vi "Test MQTT-3.8.4-5.vi"(8 "error in (no error)":errorcluster, 11 "Connection Config":refnum<class "Connection.lvclass">) -> (0 "error out":errorcluster, 3 "Connection Config dup":refnum<class "Connection.lvclass">)   [LabVIEW 2013]
uses:
  <vilib>/LabVIEW Open Source Project/MQTT Connection/MQTT_Connection/Connection/Connection.lvclass
  <vilib>/LabVIEW Open Source Project/MQTT Control Packets/Control Packets/SUBSCRIBE/Topic Subscription -- cluster.ctl
  <vilib>/LabVIEW Open Source Project/MQTT Control Packets/Control Packets/ControlPacket/QualityOfService -- enum.ctl
  <vilib>/addons/_JKI Toolkits/Caraya/classes/Test/Test.lvclass
  <vilib>/LabVIEW Open Source Project/MQTT Client/Client class/Client.lvclass
  <vilib>/LabVIEW Open Source Project/MQTT Control Packets/Control Packets/SUBSCRIBE/SUBSCRIBE.lvclass
  <vilib>/addons/_JKI Toolkits/Caraya/classes/Assert/Assert.lvclass
  <vilib>/LabVIEW Open Source Project/MQTT Connection/MQTT_Base/Base Class/MQTT_Base.lvclass
  <vilib>/LabVIEW Open Source Project/MQTT Control Packets/Control Packets/ControlPacket/ControlPacket.lvclass
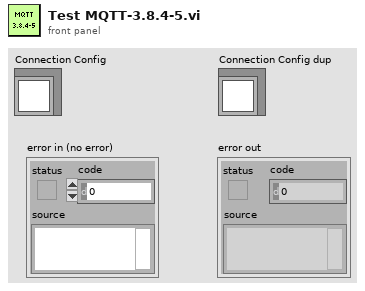
[diagram p1: front panel]
types:
  T1 = typedef "MQTT_Control_Packets.lvlib/SUBSCRIBE.lvclass/Topic Subscription -- cluster.ctl" = cluster{"Topic Filter":string, "QoS":T2}
  T2 = typedef "MQTT_Control_Packets.lvlib/ControlPacket.lvclass/QualityOfService -- enum.ctl" = enum16{"0 (At Most Once)", "1 (At Least Once)", "2 (Exactly Once)"}
  T3 = typedef "MQTT_Control_Packets.lvlib/SUBACK.lvclass/Subscription Success Code.ctl" = cluster{"Subscription Failure":bool, "QoS":T2}
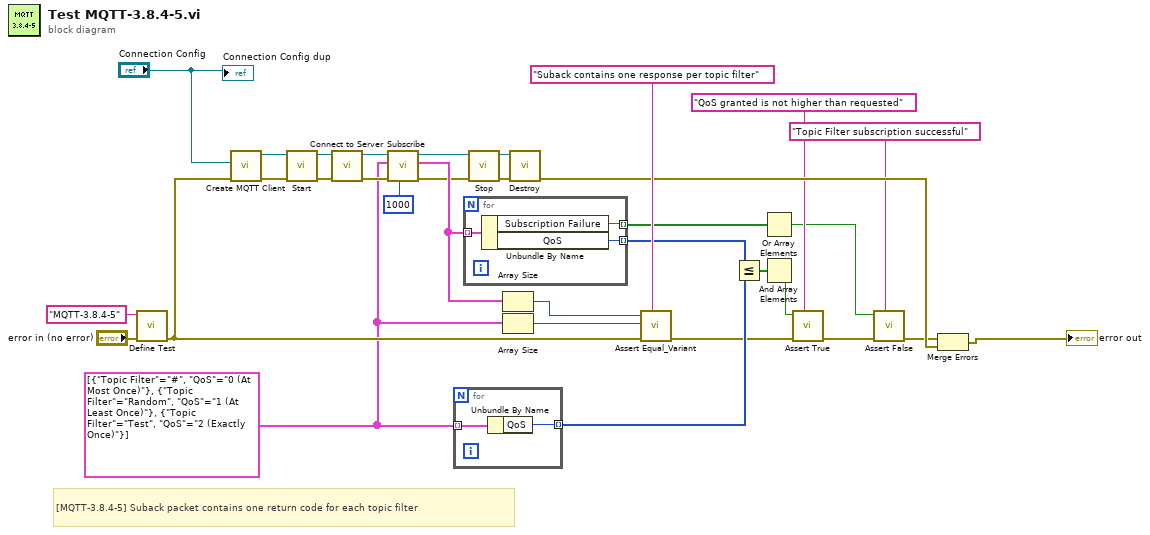
[diagram p0: block diagram]
diagram:
  w13 = T1[] [{"Topic Filter"="#", "QoS"=enum."0 (At Most Once)"}, {"Topic Filter"="Random", "QoS"=enum."1 (At Least Once)"}, {"Topic Filter"="Test", "QoS"=enum."2 (Exactly Once)"}] ("Topic Subscriptions")
  # "[MQTT-3.8.4-5] Suback packet contains one return code for each topic filter"
  n1 = call <vilib>:"Define Test.vi"("error in (no error)"="error in (no error)", "Label (VI Title)"="MQTT-3.8.4-5") -> ("error out"=w14:errorcluster)  [unwired: 9 in]
  n2 = call <vilib>:"Create MQTT Client.vi"("error in (no error)"=w14, "Connection Configuration"="Connection Config") -> ("error out"=w21:errorcluster, "Client out"=w22:refnum<class "Client.lvclass">)  [unwired: 8 in]
  n3 = call <vilib>:"Start.vi"("error in (no error)"=w21, "MQTT_Base in"=w22) -> ("error out"=w28:errorcluster, "MQTT_Base out"=w29:refnum<class "Client.lvclass">)  [unwired: 7 in, 1 out]
  n4 = call <vilib>:"Connect to Server.vi"("error in (no error)"=w28, "Client in"=w29) -> ("error out"=w24:errorcluster, "Client out"=w25:refnum<class "Client.lvclass">)  [unwired: 6 in, 2 out]
  n5 = call <vilib>:"Subscribe.vi"("timeout (1000 ms)"=1000, "error in (no error)"=w24, "Topic Subscriptions"=w13, "MQTT_Base in"=w25) -> ("error out"=w16:errorcluster, "Subscription Success"=w20:T3[], "MQTT_Base out"=w17:refnum<class "Client.lvclass">)  [unwired: 4 in, 1 out]
  n6 = for {
    tunnel: w13 -> [w35] mode=indexing
    tunnel: [w34] -> w11 mode=indexing
    n7 = Unbundle By Name(w35) -> ("QoS"=w34:T2)
  }
  n8 = for {
    tunnel: w20 -> [w38] mode=indexing
    tunnel: [w37] -> w7 mode=indexing
    tunnel: [w36] -> w12 mode=indexing
    n9 = Unbundle By Name(w38) -> ("Subscription Failure"=w37:bool, "QoS"=w36:T2)
  }
  n10 = call <vilib>:"Stop.vi"("error in (no error)"=w16, "MQTT_Base in"=w17) -> ("error out"=w26:errorcluster, "MQTT_Base out"=w27:refnum<class "Client.lvclass">)  [unwired: 7 in, 1 out]
  n11 = Array Size(array=w20) -> (size(s)=w18:i32)
  n12 = Array Size(array=w13) -> (size(s)=w19:i32)
  n13 = call <vilib>:"Destroy.vi"("error in (no error)"=w26, "MQTT_Base in"=w27) -> ("error out"=w30:errorcluster)  [unwired: 8 in, 1 out]
  n14 = call <vilib>:"Assert Equal_Variant.vi"("Label"="Suback contains one response per topic filter", "error in (no error)"=w14, "Y"=w19, "X"=w18) -> ("error out"=w2:errorcluster)  [unwired: 7 in]
  n15 = Less Or Equal?(x=w12, y=w11) -> (x <= y?=w8:bool[])
  n16 = Or Array Elements(Boolean array=w7) -> (logical OR=w4:bool)
  n17 = And Array Elements(Boolean array=w8) -> (logical AND=w10:bool)
  n18 = call <vilib>:"Assert True.vi"("Label"="QoS granted is not higher than requested", "error in (no error)"=w2, "True?"=w10) -> ("error out"=w6:errorcluster)  [unwired: 8 in]
  n19 = call <vilib>:"Assert False.vi"("Label"="Topic Filter subscription successful", "error in (no error)"=w6, "False?"=w4) -> ("error out"=w5:errorcluster)  [unwired: 8 in]
  n20 = Merge Errors(w5, w30) -> (→"error out":errorcluster)
  "Connection Config dup" <- "Connection Config"
